vi "Evaluate Part 2 attempt 2.vi"() -> ()   [LabVIEW 2020]
uses:
  a15f7c83-edd5-476e-bace-804302ff7b13.vi
  <vilib>/Comparison/Less/Less Functor/Less Functor.lvclass
  Proto/Proto.lvclass
panel:
  out "sorted array":T1(array[cluster])
  out "Numeric":i32
  out "x = y?":bool
  out "number":u64
  out "Array":bool[](array[boolean])
  in  "Input":string="x00: 1\nx01: 0\nx02: 1\nx03: 1\nx04: 0\ny00: 1\ny01: 1\ny02: 1\ny03: 1\ny04: 1\n\nntg XOR fgs -> mjb\ny02 OR x01 -> tnw\nkwq OR kpj -> z05\nx00 OR x03 -> fst\ntgd XOR rvg -> z01\nvdt OR tnw -> bfw\nbfw AND frj -> z10\nffh OR nrd -> bqk\ny00 AND y03 -> djm\ny03 OR y00 -> psh\nbqk OR frj -> z08\ntnw OR fst -> frj\ngnj AND tgd -> z11\nbfw XOR mjb -> z00\nx03 OR x00 -> vdt\ngnj AND wpb -> z02\nx04 AND y00 -> kjc\ndjm OR pbm -> qhw\nnrd AND vdt -> hwm\nkjc AND fst -> rvg\ny04 OR y02 -> fgs\ny01 AND x02 -> pbm\nntg OR kjc -> kwq\npsh XOR fgs -> tgd\nqhw XOR tgd -> z09\npbm OR djm -> kpj\nx03 XOR y03 -> ffh\nx00 XOR y04 -> ntg\nbfw OR bqk -> z06\nnrd XOR fgs -> wpb\nfrj XOR qhw -> z04\nbqk OR frj -> z07\ny03 OR x01 -> nrd\nhwm AND bqk -> z03\ntgd XOR rvg -> z12\ntnw OR pbm -> gnj"
  # "2947015374 too low\n\n282578783305985 too high\n66055249060558"
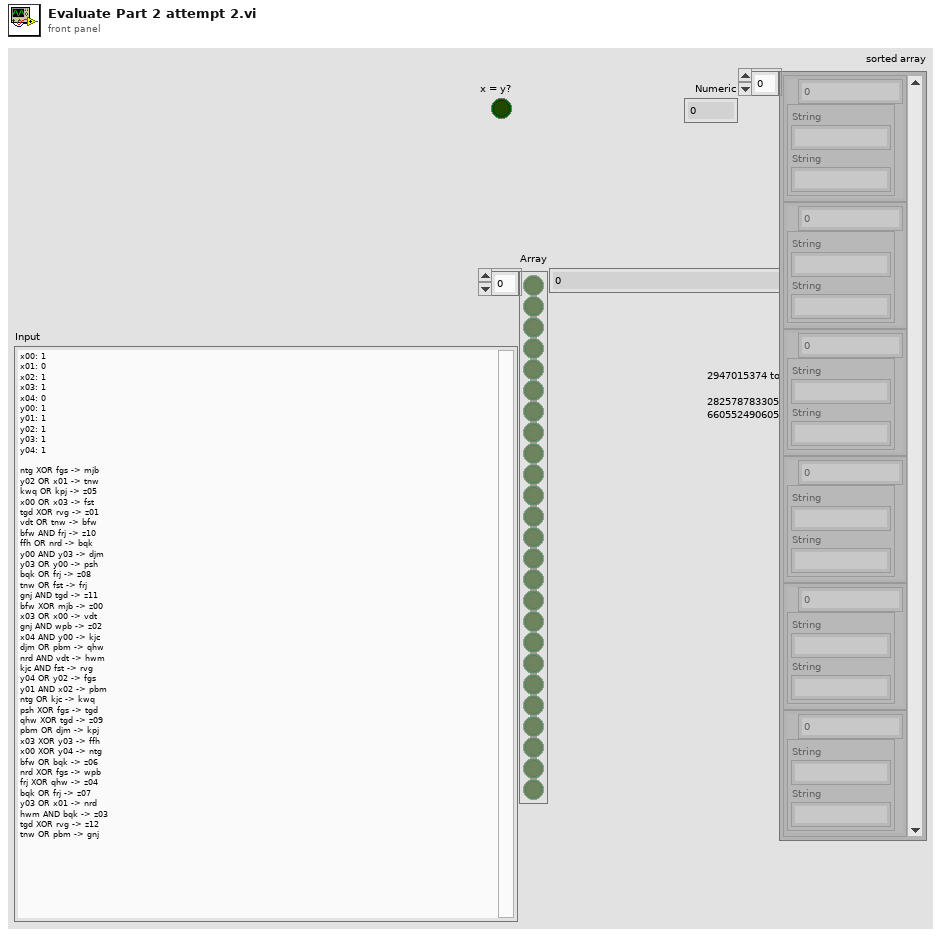
[diagram p1: front panel]
types:
  T1 = cluster{u64, cluster{"String":string, "String":string}}[]
  T2 = cluster{u64, cluster{"String":string, "String":string}}
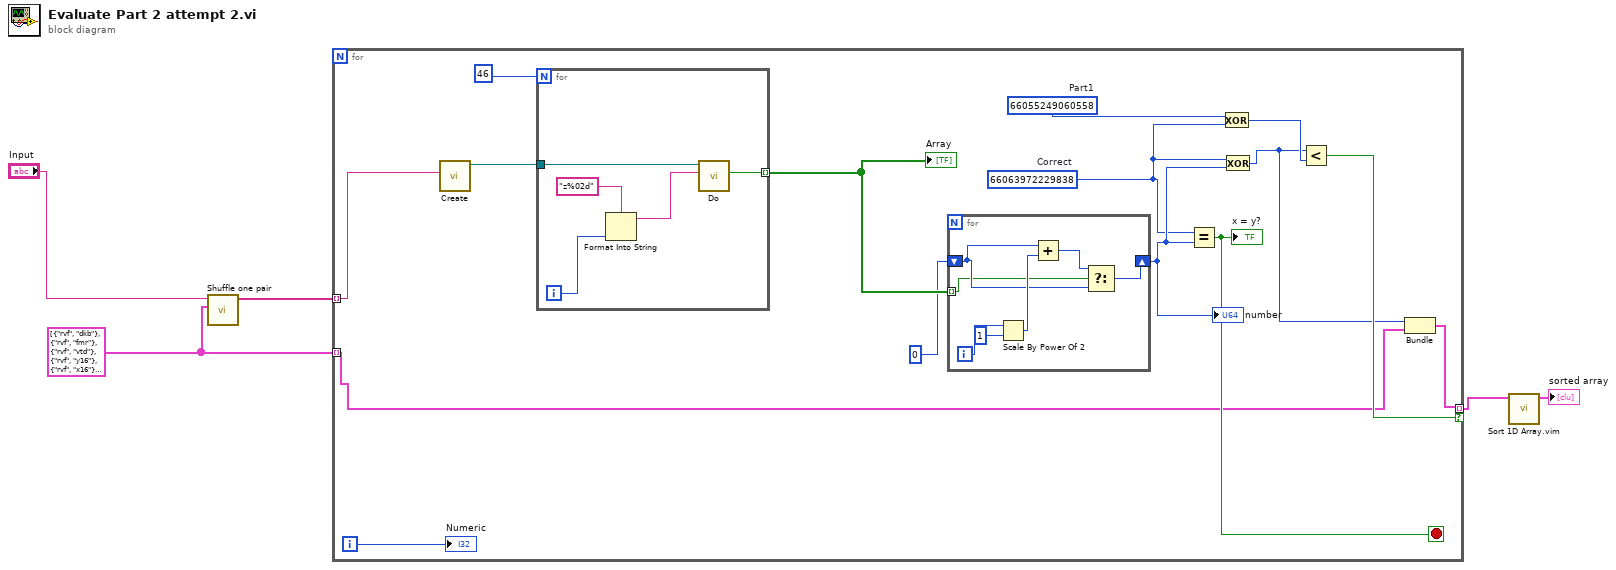
[diagram p0: block diagram]
diagram:
  w3 = cluster{"String":string, "String":string}[] [{"String"="rvf", "String"="dkb"}, {"String"="rvf", "String"="fmr"}, {"String"="rvf", "String"="vtd"}, {"String"="rvf", "String"="y16"}, {"String"="rvf", "String"="x16"}, {"String"="rvf", "String"="gdq"}, {"String"="rvf", "String"="chf"}, {"String"="rvf", "String"="krw"}, {"String"="rvf", "String"="vnk"}, {"String"="rvf", "String"="mvn"}, {"String"="rvf", "String"="wjt"}, {"String"="rvf", "String"="dtn"}, {"String"="rvf", "String"="ntn"}, {"String"="rvf", "String"="wkw"}, {"String"="rvf", "String"="jgr"}, {"String"="rvf", "String"="fcd"}, {"String"="rvf", "String"="mgc"}, {"String"="rvf", "String"="pns"}, {"String"="rvf", "String"="tsc"}, {"String"="dkb", "String"="fmr"}, {"String"="dkb", "String"="vtd"}, {"String"="dkb", "String"="y16"}, {"String"="dkb", "String"="x16"}, {"String"="dkb", "String"="gdq"}, {"String"="dkb", "String"="chf"}, {"String"="dkb", "String"="krw"}, {"String"="dkb", "String"="vnk"}, {"String"="dkb", "String"="mvn"}, {"String"="dkb", "String"="wjt"}, {"String"="dkb", "String"="dtn"}, {"String"="dkb", "String"="ntn"}, {"String"="dkb", "String"="wkw"}, {"String"="dkb", "String"="jgr"}, {"String"="dkb", "String"="fcd"}, {"String"="dkb", "String"="mgc"}, {"String"="dkb", "String"="pns"}, {"String"="dkb", "String"="tsc"}, {"String"="fmr", "String"="vtd"}, {"String"="fmr", "String"="y16"}, {"String"="fmr", "String"="x16"}, {"String"="fmr", "String"="gdq"}, {"String"="fmr", "String"="chf"}, {"String"="fmr", "String"="krw"}, {"String"="fmr", "String"="vnk"}, {"String"="fmr", "String"="mvn"}, {"String"="fmr", "String"="wjt"}, {"String"="fmr", "String"="dtn"}, {"String"="fmr", "String"="ntn"}, {"String"="fmr", "String"="wkw"}, {"String"="fmr", "String"="jgr"}, {"String"="fmr", "String"="fcd"}, {"String"="fmr", "String"="mgc"}, {"String"="fmr", "String"="pns"}, {"String"="fmr", "String"="tsc"}, {"String"="vtd", "String"="y16"}, {"String"="vtd", "String"="x16"}, {"String"="vtd", "String"="gdq"}, {"String"="vtd", "String"="chf"}, {"String"="vtd", "String"="krw"}, {"String"="vtd", "String"="vnk"}, {"String"="vtd", "String"="mvn"}, {"String"="vtd", "String"="wjt"}, {"String"="vtd", "String"="dtn"}, {"String"="vtd", "String"="ntn"}, {"String"="vtd", "String"="wkw"}, {"String"="vtd", "String"="jgr"}, {"String"="vtd", "String"="fcd"}, {"String"="vtd", "String"="mgc"}, {"String"="vtd", "String"="pns"}, {"String"="vtd", "String"="tsc"}, {"String"="y16", "String"="x16"}, {"String"="y16", "String"="gdq"}, {"String"="y16", "String"="chf"}, {"String"="y16", "String"="krw"}, {"String"="y16", "String"="vnk"}, {"String"="y16", "String"="mvn"}, {"String"="y16", "String"="wjt"}, {"String"="y16", "String"="dtn"}, {"String"="y16", "String"="ntn"}, {"String"="y16", "String"="wkw"}, {"String"="y16", "String"="jgr"}, {"String"="y16", "String"="fcd"}, {"String"="y16", "String"="mgc"}, {"String"="y16", "String"="pns"}, {"String"="y16", "String"="tsc"}, {"String"="x16", "String"="gdq"}, {"String"="x16", "String"="chf"}, {"String"="x16", "String"="krw"}, {"String"="x16", "String"="vnk"}, {"String"="x16", "String"="mvn"}, {"String"="x16", "String"="wjt"}, {"String"="x16", "String"="dtn"}, {"String"="x16", "String"="ntn"}, {"String"="x16", "String"="wkw"}, {"String"="x16", "String"="jgr"}, {"String"="x16", "String"="fcd"}, {"String"="x16", "String"="mgc"}, {"String"="x16", "String"="pns"}, {"String"="x16", "String"="tsc"}, {"String"="gdq", "String"="chf"}, {"String"="gdq", "String"="krw"}, {"String"="gdq", "String"="vnk"}, {"String"="gdq", "String"="mvn"}, {"String"="gdq", "String"="wjt"}, {"String"="gdq", "String"="dtn"}, {"String"="gdq", "String"="ntn"}, {"String"="gdq", "String"="wkw"}, {"String"="gdq", "String"="jgr"}, {"String"="gdq", "String"="fcd"}, {"String"="gdq", "String"="mgc"}, {"String"="gdq", "String"="pns"}, {"String"="gdq", "String"="tsc"}, {"String"="chf", "String"="krw"}, {"String"="chf", "String"="vnk"}, {"String"="chf", "String"="mvn"}, {"String"="chf", "String"="wjt"}, {"String"="chf", "String"="dtn"}, {"String"="chf", "String"="ntn"}, {"String"="chf", "String"="wkw"}, {"String"="chf", "String"="jgr"}, {"String"="chf", "String"="fcd"}, {"String"="chf", "String"="mgc"}, {"String"="chf", "String"="pns"}, {"String"="chf", "String"="tsc"}, {"String"="krw", "String"="vnk"}, {"String"="krw", "String"="mvn"}, {"String"="krw", "String"="wjt"}, {"String"="krw", "String"="dtn"}, {"String"="krw", "String"="ntn"}, {"String"="krw", "String"="wkw"}, {"String"="krw", "String"="jgr"}, {"String"="krw", "String"="fcd"}, {"String"="krw", "String"="mgc"}, {"String"="krw", "String"="pns"}, {"String"="krw", "String"="tsc"}, {"String"="vnk", "String"="mvn"}, {"String"="vnk", "String"="wjt"}, {"String"="vnk", "String"="dtn"}, {"String"="vnk", "String"="ntn"}, {"String"="vnk", "String"="wkw"}, {"String"="vnk", "String"="jgr"}, {"String"="vnk", "String"="fcd"}, {"String"="vnk", "String"="mgc"}, {"String"="vnk", "String"="pns"}, {"String"="vnk", "String"="tsc"}, {"String"="mvn", "String"="wjt"}, {"String"="mvn", "String"="dtn"}, {"String"="mvn", "String"="ntn"}, {"String"="mvn", "String"="wkw"}, {"String"="mvn", "String"="jgr"}, {"String"="mvn", "String"="fcd"}, {"String"="mvn", "String"="mgc"}, {"String"="mvn", "String"="pns"}, {"String"="mvn", "String"="tsc"}, {"String"="wjt", "String"="dtn"}, {"String"="wjt", "String"="ntn"}, {"String"="wjt", "String"="wkw"}, {"String"="wjt", "String"="jgr"}, {"String"="wjt", "String"="fcd"}, {"String"="wjt", "String"="mgc"}, {"String"="wjt", "String"="pns"}, {"String"="wjt", "String"="tsc"}, {"String"="dtn", "String"="ntn"}, {"String"="dtn", "String"="wkw"}, {"String"="dtn", "String"="jgr"}, {"String"="dtn", "String"="fcd"}, {"String"="dtn", "String"="mgc"}, {"String"="dtn", "String"="pns"}, {"String"="dtn", "String"="tsc"}, {"String"="ntn", "String"="wkw"}, {"String"="ntn", "String"="jgr"}, {"String"="ntn", "String"="fcd"}, {"String"="ntn", "String"="mgc"}, {"String"="ntn", "String"="pns"}, {"String"="ntn", "String"="tsc"}, {"String"="wkw", "String"="jgr"}, {"String"="wkw", "String"="fcd"}, {"String"="wkw", "String"="mgc"}, {"String"="wkw", "String"="pns"}, {"String"="wkw", "String"="tsc"}, {"String"="jgr", "String"="fcd"}, {"String"="jgr", "String"="mgc"}, {"String"="jgr", "String"="pns"}, {"String"="jgr", "String"="tsc"}, {"String"="fcd", "String"="mgc"}, {"String"="fcd", "String"="pns"}, {"String"="fcd", "String"="tsc"}, {"String"="mgc", "String"="pns"}, {"String"="mgc", "String"="tsc"}, {"String"="pns", "String"="tsc"}] ("Array")
  n1 = call "Shuffle one pair.vi"("Array in"=w3, "Input"="Input") -> ("Array out"=w4:string[])  [unwired: 9 in]
  n2 = for {
    tunnel: w4 -> [w9] mode=indexing
    tunnel: [w6] -> w2 mode=indexing if=w10
    tunnel: w3 -> [w8] mode=indexing
    i -> [w15]
    stop <- w16 stop-if-true
    w13 = u64 66055249060558  # Part1
    w12 = u64 66063972229838  # Correct
    n3 = call "Create.vi"("Input"=w9) -> ("Proto"=w20:refnum<class "Proto.lvclass">)  [unwired: 9 in, 1 out]
    n4 = for {
      N: 46 -> [_]
      tunnel: w20 -> [w25]
      tunnel: [w21] -> w19 mode=indexing
      i -> [w23]
      n5 = Format Into String(format string="z%02d", w23) -> (resulting string=w22:string)  [unwired: 2 in, 1 out]
      n6 = call "Do.vi"("Key"=w22, "Proto in"=w25) -> ("Value"=w21:bool)  [unwired: 7 in, 2 out]
    }
    "Array" <- w19
    n7 = for {
      tunnel: w19 -> [w28] mode=indexing
      shift-right: [w26] -> w14
      shift-left: u64 0 ("number") -> [w29]
      i -> [w32]
      n8 = Scale By Power Of 2(n=w32, x=u64 1) -> (x*2^n=w30:u64)
      n9 = Add(x=w29, y=w30) -> (x+y=w27:u64)
      n10 = Select(t=w27, s=w28, f=w29) -> (s? t:f=w26:u64)
    }
    "number" <- w14
    n11 = Equal?(x=w12, y=w14) -> (x = y?=w16:bool)
    "x = y?" <- w16
    n12 = Exclusive Or(1:w12, 2:w13) -> (0:w11:u64)
    n13 = Exclusive Or(1:w14, 2:w12) -> (0:w7:u64)
    n14 = Less?(x=w7, y=w11) -> (x < y?=w10:bool)
    n15 = Bundle(w7, w8) -> (w6:T2)  [unwired: 1 in]
    "Numeric" <- w15
  }
  n16 = call "Sort 1D Array.vim"("unsorted array"=w2) -> ("sorted array"=→"sorted array":T1)  [unwired: 10 in]
